vi "Populate Menu Items.vi"(8 "Error In":errorcluster, 9 "ClearOldMenus (T)":bool=TRUE, 10 "MenuHierarchyPaths":string[](array[string]), 11 "MenuRef":refnum<k9>) -> (0 "Error Out":errorcluster)   [LabVIEW 2016, in "SLL Menu.lvlib"]
doc: "Takes a runtime MenuRef and an array of colon-delimited path strings, then during the Shortcut Menu Activation event, builds (or reuses) each hierarchical level by checking if a full-path tag exists and inserting missing items under their parent so the shortcut menu reflects the requested structure."
uses:
  SLL Menu.lvlib
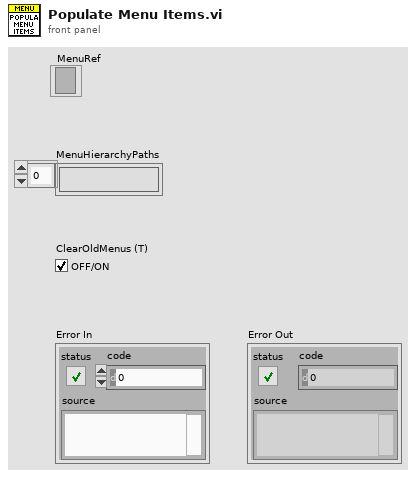
[diagram p1: front panel]
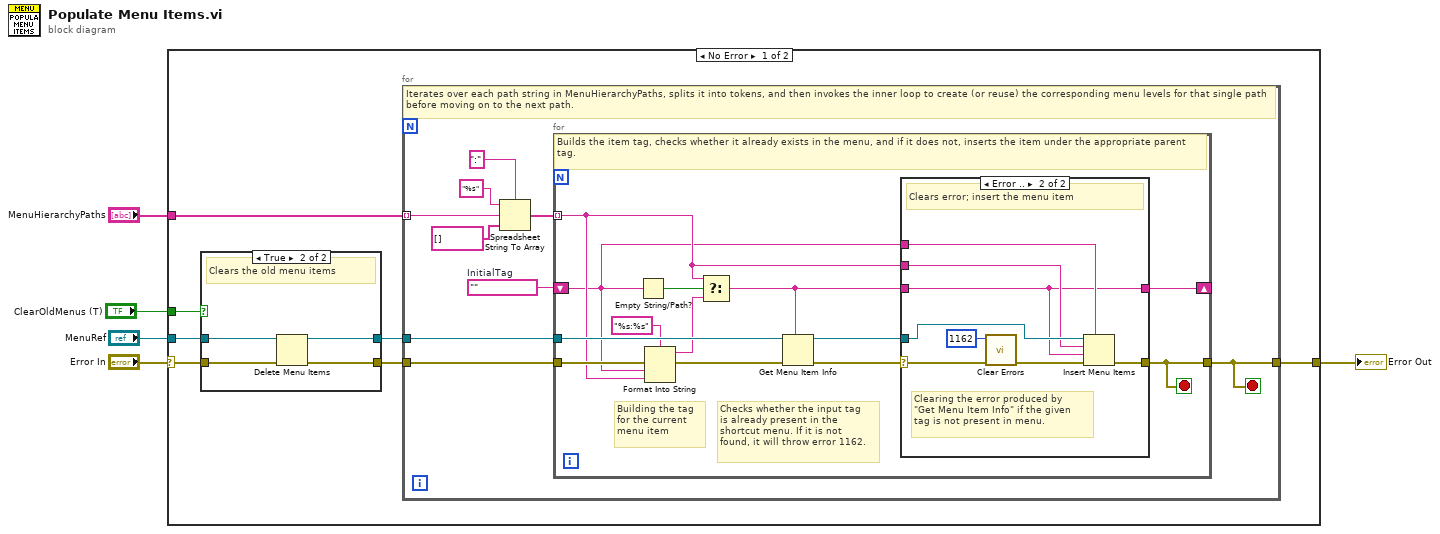
[diagram p0: block diagram]
diagram:
  n1 = case shown="No Error" "Error In" {
    selector: "Error In" -> [w12 w51]
    tunnel: "MenuRef" -> [w10 _]
    tunnel: [w8 w51] -> w4
    tunnel: "MenuHierarchyPaths" -> [w7 _]
    tunnel: "ClearOldMenus (T)" -> [w6 _]
    frame No Error {
      n2 = case shown="True" w6 {
        tunnel: w12 -> [w14 w18]
        tunnel: [w14 w17] -> w11
        tunnel: w10 -> [w13 w16]
        tunnel: [w13 w15] -> w9
        frame False {
          # "Passes the menu reference and error wire without any changes"
        }
        frame True {
          # "Clears the old menu items"
          n3 = Delete Menu Items(6:w18, 9:w16) -> (0:w17:errorcluster, 3:w15:refnum<k9>)  [unwired: 2 in]
        }
      }
      n4 = for {
        tunnel: w9 -> [w19]
        tunnel: w7 -> [w24] mode=indexing
        tunnel: w11 -> [w27]
        tunnel: [w22] -> w8
        stop <- w22 stop-if-true
        w20 = ""  # InitialTag
        # "Iterates over each path string in MenuHierarchyPaths, splits it into tokens, and then invokes the inner loop to create (or reuse) the corresponding menu levels for that single path before moving on to the next path."
        n5 = Spreadsheet String To Array(delimiter (Tab)=":", format string="%s", spreadsheet string=w24, array type (2D Dbl)=string[] []) -> (array=w21:string[])
        n6 = for {
          tunnel: w21 -> [w32] mode=indexing
          shift-right: [w36] -> _
          shift-left: w20 -> [w29]
          tunnel: w19 -> [w38]
          tunnel: w27 -> [w40]
          tunnel: [w28] -> w22
          stop <- w28 stop-if-true
          # "Checks whether the input tag \nis already present in the \nshortcut menu. If it is not \nfound, it will throw error 1162."
          # "Building the tag \nfor the current \nmenu item"
          # "Builds the item tag, checks whether it already exists in the menu, and if it does not, inserts the item under the appropriate parent tag."
          n7 = Empty String/Path?(string/path=w29) -> (empty?=w35:bool)
          n8 = Format Into String(format string="%s:%s", error in=w40, w29, w32) -> (resulting string=w30:string, error out=w33:errorcluster)  [unwired: 1 in]
          n9 = Select(t=w32, s=w35, f=w30) -> (s? t:f=w34:string)
          n10 = Get Menu Item Info(7:w34, 8:w33, 11:w38) -> (0:w39:errorcluster, 3:w37:refnum<k9>)  [unwired: 5 out]
          n11 = case shown="Error .." w39 {
            selector: w39 -> [w42 w50]
            tunnel: [w42 w48] -> w28
            tunnel: w37 -> [_ w47]
            tunnel: w29 -> [_ w46]
            tunnel: w34 -> [w41 w44]
            tunnel: w32 -> [_ w45]
            tunnel: [w41 w44] -> w36
            frame No Error {
              # "Does nothing, as the item already exists in the menu."
            }
            frame Error {
              # "Clearing the error produced by \n\"Get Menu Item Info\" if the given \ntag is not present in menu."
              # "Clears error; insert the menu item"
              n12 = call <vilib>:"Clear Errors.vi"("error in (no error)"=w50, "specific error code to clear (0: all)"=1162) -> ("error out"=w49:errorcluster)  [unwired: 4 in, 1 out]
              n13 = Insert Menu Items(5:w46, 6:w49, 7:w44, 8:w45, 9:w47) -> (0:w48:errorcluster)  [unwired: 1 in, 2 out]
            }
          }
        }
      }
    }
    frame Error {
    }
  }
  "Error Out" <- w4
